vi "ground_pressure_data_parser.vi"() -> ()   [LabVIEW 2020]
uses:
  <vilib>/Utility/file.llb/Read Delimited Spreadsheet (string).vi
panel:
  out "Array":dbl[][](array[numeric])
  out "all rows":string[][](array[string])
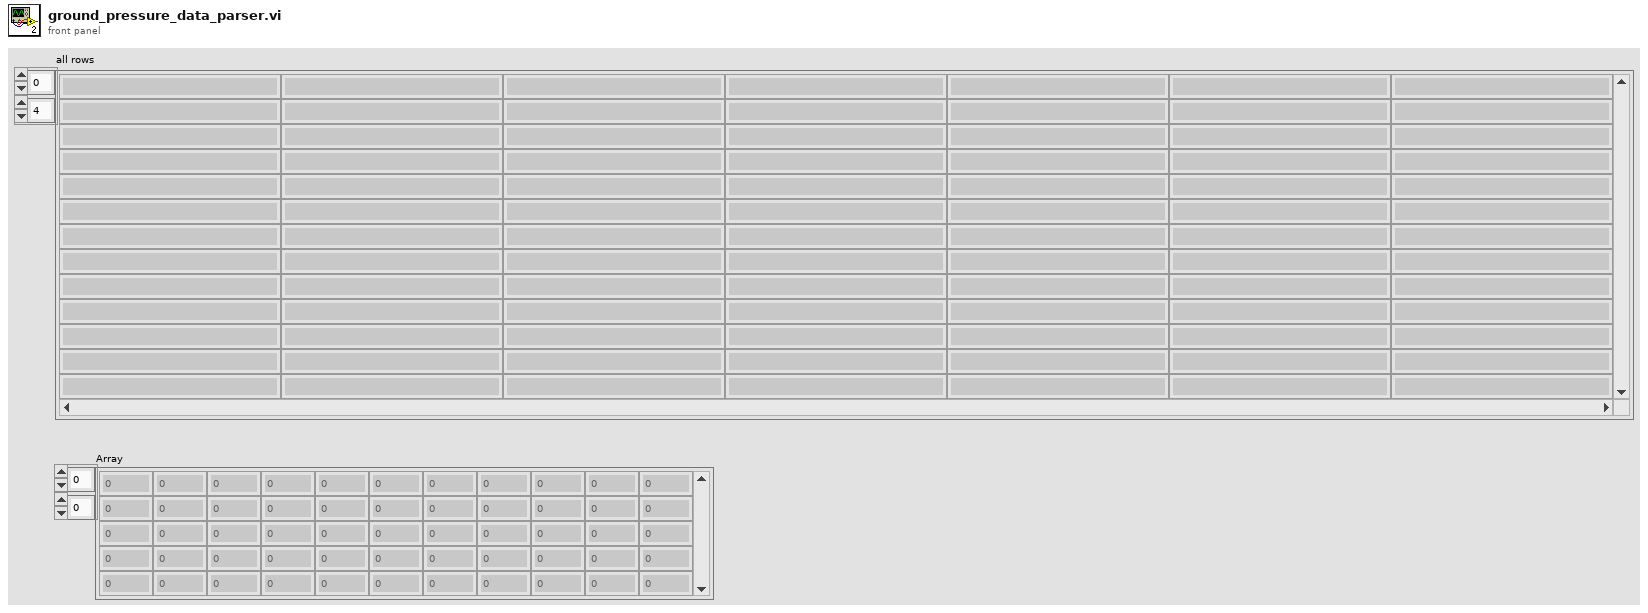
[diagram p1: front panel]
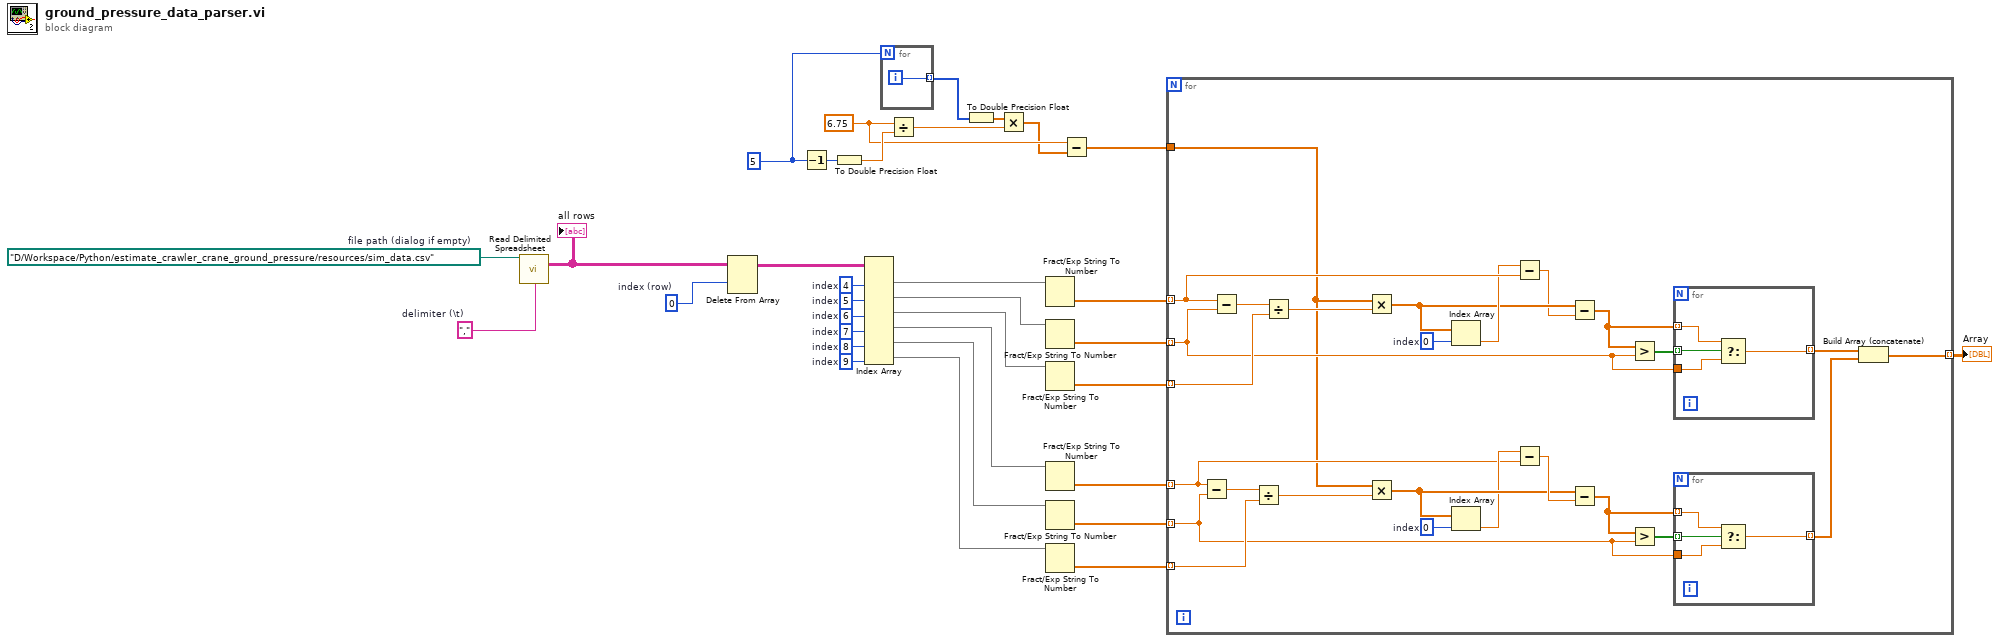
[diagram p0: block diagram]
diagram:
  w9 = 5
  w4 = 6.75
  w23 = 9  # index
  w24 = 8  # index
  w25 = 7  # index
  w26 = 6  # index
  w27 = 5  # index
  w28 = 4  # index
  w30 = 0  # index (row)
  w32 = ","  # delimiter (\t)
  w33 = path "D:/Workspace/Python/estimate_crawler_crane_ground_pressure/resources/sim_data.csv"  # file path (dialog if empty)
  n1 = call-poly <vilib>:"Read Delimited Spreadsheet.vi"("file path (dialog if empty)"=w33, "delimiter (\\t)"=w32) -> ("all rows"=w31:string[][])  [unwired: 8 in, 5 out]
  "all rows" <- w31
  n2 = Delete From Array(array=w31, index (row)=w30) -> (array with subset deleted=w29:string[][])  [unwired: 2 in, 1 out]
  n3 = Decrement(x=w9) -> (x-1=w10:i32)
  n4 = To Double Precision Float(number=w10) -> (double precision float=w8:dbl)
  n5 = Index Array(array=w29, index (col) #1=w28, index (col) #2=w27, index (col) #3=w26, index (col) #4=w25, index (col) #5=w24, index (col) #6=w23) -> (element #1=w22:string[], element #2=w21:string[], element #3=w20:string[], element #4=w19:string[], element #5=w18:string[], element #6=w17:string[])  [unwired: 6 in]
  n6 = for {
    N: w9 -> [_]
    tunnel: [w34] -> w7 mode=indexing
    i -> [w34]
  }
  n7 = Divide(x=w4, y=w8) -> (x/y=w5:dbl)
  n8 = To Double Precision Float(number=w7) -> (double precision float=w6:dbl[])
  n9 = Multiply(x=w6, y=w5) -> (x*y=w3:dbl[])
  n10 = Fract/Exp String To Number(string=w22) -> (number=w16:dbl[])  [unwired: 3 in, 1 out]
  n11 = Fract/Exp String To Number(string=w21) -> (number=w15:dbl[])  [unwired: 3 in, 1 out]
  n12 = Fract/Exp String To Number(string=w20) -> (number=w14:dbl[])  [unwired: 3 in, 1 out]
  n13 = Fract/Exp String To Number(string=w19) -> (number=w13:dbl[])  [unwired: 3 in, 1 out]
  n14 = Fract/Exp String To Number(string=w18) -> (number=w12:dbl[])  [unwired: 3 in, 1 out]
  n15 = Fract/Exp String To Number(string=w17) -> (number=w11:dbl[])  [unwired: 3 in, 1 out]
  n16 = Subtract(x=w4, y=w3) -> (x-y=w2:dbl[])
  n17 = for {
    tunnel: w16 -> [w54] mode=indexing
    tunnel: w15 -> [w48] mode=indexing
    tunnel: w14 -> [w57] mode=indexing
    tunnel: w13 -> [w41] mode=indexing
    tunnel: w12 -> [w40] mode=indexing
    tunnel: w11 -> [w58] mode=indexing
    tunnel: w2 -> [w38]
    tunnel: [w35] -> w1 mode=indexing
    w42 = 0  # index
    w55 = 0  # index
    n18 = Subtract(x=w41, y=w40) -> (x-y=w59:dbl)
    n19 = Subtract(x=w54, y=w48) -> (x-y=w60:dbl)
    n20 = Divide(x=w59, y=w58) -> (x/y=w39:dbl)
    n21 = Divide(x=w60, y=w57) -> (x/y=w56:dbl)
    n22 = Multiply(x=w38, y=w56) -> (x*y=w52:dbl[])
    n23 = Multiply(x=w38, y=w39) -> (x*y=w44:dbl[])
    n24 = Index Array(array=w52, index=w55) -> (element=w53:dbl)
    n25 = Index Array(array=w44, index=w42) -> (element=w43:dbl)
    n26 = Subtract(x=w53, y=w54) -> (x-y=w51:dbl)
    n27 = Subtract(x=w43, y=w41) -> (x-y=w45:dbl)
    n28 = Subtract(x=w52, y=w51) -> (x-y=w49:dbl[])
    n29 = Subtract(x=w44, y=w45) -> (x-y=w47:dbl[])
    n30 = Greater?(x=w49, y=w48) -> (0:w50:bool[])
    n31 = Greater?(x=w47, y=w40) -> (0:w46:bool[])
    n32 = for {
      tunnel: w50 -> [w68] mode=indexing
      tunnel: w49 -> [w67] mode=indexing
      tunnel: w48 -> [w66]
      tunnel: [w65] -> w37 mode=indexing
      n33 = Select(t=w67, s=w68, f=w66) -> (s? t:f=w65:dbl)
    }
    n34 = for {
      tunnel: w46 -> [w64] mode=indexing
      tunnel: w47 -> [w63] mode=indexing
      tunnel: w40 -> [w62]
      tunnel: [w61] -> w36 mode=indexing
      n35 = Select(t=w63, s=w64, f=w62) -> (s? t:f=w61:dbl)
    }
    n36 = Build Array (concatenate)(w37, w36) -> (w35:dbl[])
  }
  "Array" <- w1
